vi "moveZ_Sutter.vi"(0 "Z":dbl format="%0.2f") -> ()   [LabVIEW 2015]
uses:
  Zstack2/XYZStage/XYZStage State.ctl
  Zstack2/XYZStage/XYZStage Loop State.ctl
  Zstack2/XYZStage/XYZStage.lvlib
panel:
  in  "Hardware State":T1
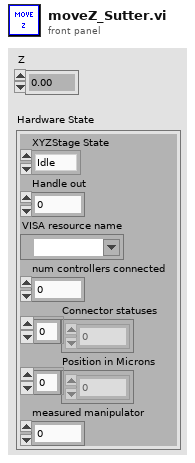
[diagram p1: front panel]
types:
  T1 = typedef "XYZStage.lvlib/XYZStage State.ctl" = cluster{"XYZStage State":T2, "Handle out":u32, "VISA resource name":refnum<visa-resource-name>, "num controllers connected":u8, "Connector statuses":u8[], "Position in Microns":dbl[], "measured manipulator":u8}
  T2 = typedef "XYZStage.lvlib/XYZStage Loop State.ctl" = enum16{"Idle", "Connected", "Moving"}
  T3 = typedef "XYZStage.lvlib/XYZStage Configuration.ctl" = cluster{"VISA resource name":refnum<visa-resource-name>, "Timeout (3sec)":u32}
  T4 = cluster{"StageS":i32, "StageL":i32, "currmeas data dir":path, "image OD":u16, "contour OD":u16, "point OD":u16, "AOlines":tag[], "AIlines":tag[], "CI lines":tag[], "DO lines":tag[], "AO names":string[], "CI names":string[], "AI names":string[], "DO names":string[], "CIextensions":string[], "AIextensions":string[], "Voltage to Ygalvo":i32, "Voltage to Xgalvo":i32, "Voltage to patch":i32, "640 shutter":i32, "2P shutter":i32, "LT timestamp":u32, "Vp":i32, "Ip":i32, "camera trigger":i32, "master data dir":path, "voltage to Zpos":i32, "Vto2P":i32, "640 AO":i32, "488 AO":i32, "532 AO":i32, "640TTL":u32, "488TTL":u32, "532TTL":u32, "Device 1 sampleclock out":tag, "Device 1 Starttrigger out":tag, "Device 2 sampleclock in":tag, "Device 2 StartTrigger in ":tag, "2PODTTL":u32, "488 shutter":u32, "LCVR red":u32, "LCVR blue":u32, "Sutter Stage Config":T3, "Device 1 ext sampleclock in (100Khz)":tag}
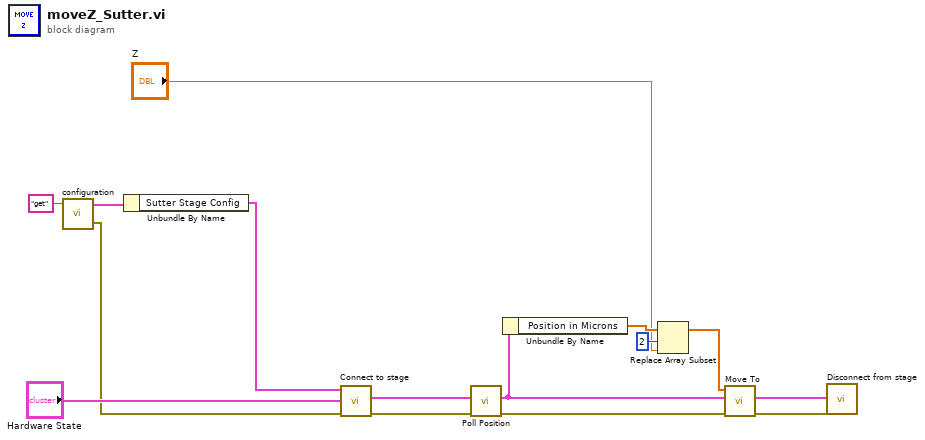
[diagram p0: block diagram]
diagram:
  n1 = call "configuration.vi"("command"="get") -> ("Error out"=w3:errorcluster, "config out"=w2:T4)  [unwired: 2 in]
  n2 = Unbundle By Name(w2) -> ("Sutter Stage Config"=w1:T3)
  n3 = call "Connect to stage.vi"("error in (no error)"=w3, "Hardware State"="Hardware State", "Hardware Configuration"=w1) -> ("error out"=w13:errorcluster, "Hardware State Out"=w14:T1)  [unwired: 6 in, 1 out]
  n4 = call "Poll Position.vi"("error in (no error)"=w13, "Hardware State"=w14) -> ("error out"=w12:errorcluster, "Hardware State Out"=w9:T1)  [unwired: 7 in, 1 out]
  n5 = Unbundle By Name(w9) -> ("Position in Microns"=w8:dbl[])
  n6 = Replace Array Subset(array=w8, new element="Z", index=2) -> (w5:dbl[])
  n7 = call "Move To.vi"("error in (no error)"=w12, "Hardware State"=w9, "New Position"=w5) -> ("error out"=w11:errorcluster, "Hardware State Out"=w10:T1)  [unwired: 7 in]
  n8 = call "Disconnect from stage.vi"("error in (no error)"=w11, "Hardware State"=w10) -> ()  [unwired: 8 in, 2 out]
